vi "ListBox Demo.vi"() -> ()   [LabVIEW 2020]
uses:
  AutoComplete/AutoComplete.lvlib
panel:
  in  "Autohide List?":bool
  in  "Listbox":i32(listbox)
  out "Selection":string
  in  "String":string
  # "This example uses an existing listbox that's part of this VI to show the filtered items."
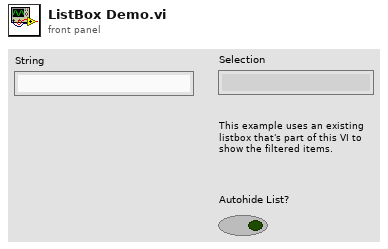
[diagram p1: front panel]
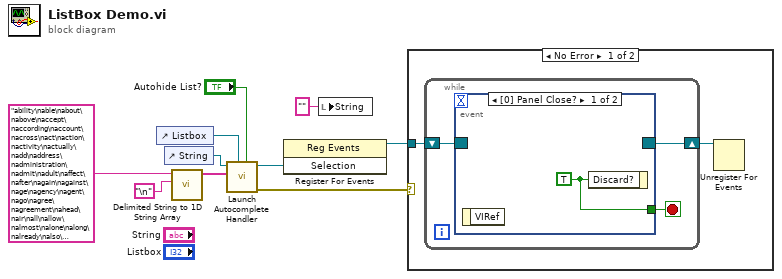
[diagram p0: block diagram]
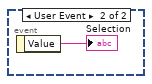
[diagram p2: hidden frame]
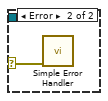
[diagram p3: hidden frame]
diagram:
  n1 = control-ref of="Listbox"() -> (w6:refnum<vi>)
  n2 = control-ref of="String"() -> (w7:refnum<vi>)
  n3 = call <vilib>:"Delimited String to 1D String Array.vi"("delimiter"="\n", "delimited string"="ability\nable\nabout\nabove\naccept\naccording\naccount\nacross\nact\naction\nactivity\nactually\nadd\naddress\nadministration\nadmit\nadult\naffect\nafter\nagain\nagainst\nage\nagency\nagent\nago\nagree\nagreement\nahead\nair\nall\nallow\nalmost\nalone\nalong\nalready\nalso\nalthough\nalways\nAmerican\namong\namount\nanalysis\nand\nanimal\nanother\nanswer\nany\nanyone\nanything\nappear\napply\napproach\narea\nargue\narm\naround\narrive\nart\narticle\nartist\nas\nask\nassume\nat\nattack\nattention\nattorney\naudience\nauthor\nauthority\navailable\navoid\naway\nbaby\nback\nbad\nbag\nball\nbank\nbar\nbase\nbe\nbeat\nbeautiful\nbecause\nbecome\nbed\nbefore\nbegin\nbehavior\nbehind\nbelieve\nbenefit\nbest\nbetter\nbetween\nbeyond\nbig\nbill\nbillion\nbit\nblack\nblood\nblue\nboard\nbody\nbook\nborn\nboth\nbox\nboy\nbreak\nbring\nbrother\nbudget\nbuild\nbuilding\nbusiness\nbut\nbuy\nby\ncall\ncamera\ncampaign\ncan\ncancer\ncandidate\ncapital\ncar\ncard\ncare\ncareer\ncarry\ncase\ncatch\ncause\ncell\ncenter\ncentral\ncentury\ncertain\ncertainly\nchair\nchallenge\nchance\nchange\ncharacter\ncharge\ncheck\nchild\nchoice\nchoose\nchurch\ncitizen\ncity\ncivil\nclaim\nclass\nclear\nclearly\nclose\ncoach\ncold\ncollection\ncollege\ncolor\ncome\ncommercial\ncommon\ncommunity\ncompany\ncompare\ncomputer\nconcern\ncondition\nconference\nCongress\nconsider\nconsumer\ncontain\ncontinue\ncontrol\ncost\ncould\ncountry\ncouple\ncourse\ncourt\ncover\ncreate\ncrime\ncultural\nculture\ncup\ncurrent\ncustomer\ncut\ndark\ndata\ndaughter\nday\ndead\ndeal\ndeath\ndebate\ndecade\ndecide\ndecision\ndeep\ndefense\ndegree\nDemocrat\ndemocratic\ndescribe\ndesign\ndespite\ndetail\ndetermine\ndevelop\ndevelopment\ndie\ndifference\ndifferent\ndifficult\ndinner\ndirection\ndirector\ndiscover\ndiscuss\ndiscussion\ndisease\ndo\ndoctor\ndog\ndoor\ndown\ndraw\ndream\ndrive\ndrop\ndrug\nduring\neach\nearly\neast\neasy\neat\neconomic\neconomy\nedge\neducation\neffect\neffort\neight\neither\nelection\nelse\nemployee\nend\nenergy\nenjoy\nenough\nenter\nentire\nenvironment\nenvironmental\nespecially\nestablish\neven\nevening\nevent\never\nevery\neverybody\neveryone\neverything\nevidence\nexactly\nexample\nexecutive\nexist\nexpect\nexperience\nexpert\nexplain\neye\nface\nfact\nfactor\nfail\nfall\nfamily\nfar\nfast\nfather\nfear\nfederal\nfeel\nfeeling\nfew\nfield\nfight\nfigure\nfill\nfilm\nfinal\nfinally\nfinancial\nfind\nfine\nfinger\nfinish\nfire\nfirm\nfirst\nfish\nfive\nfloor\nfly\nfocus\nfollow\nfood\nfoot\nfor\nforce\nforeign\nforget\nform\nformer\nforward\nfour\nfree\nfriend\nfrom\nfront\nfull\nfund\nfuture\ngame\ngarden\ngas\ngeneral\ngeneration\nget\ngirl\ngive\nglass\ngo\ngoal\ngood\ngovernment\ngreat\ngreen\nground\ngroup\ngrow\ngrowth\nguess\ngun\nguy\nhair\nhalf\nhand\nhang\nhappen\nhappy\nhard\nhave\nhe\nhead\nhealth\nhear\nheart\nheat\nheavy\nhelp\nher\nhere\nherself\nhigh\nhim\nhimself\nhis\nhistory\nhit\nhold\nhome\nhope\nhospital\nhot\nhotel\nhour\nhouse\nhow\nhowever\nhuge\nhuman\nhundred\nhusband\nI\nidea\nidentify\nif\nimage\nimagine\nimpact\nimportant\nimprove\nin\ninclude\nincluding\nincrease\nindeed\nindicate\nindividual\nindustry\ninformation\ninside\ninstead\ninstitution\ninterest\ninteresting\ninternational\ninterview\ninto\ninvestment\ninvolve\nissue\nit\nitem\nits\nitself\njob\njoin\njust\nkeep\nkey\nkid\nkill\nkind\nkitchen\nknow\nknowledge\nland\nlanguage\nlarge\nlast\nlate\nlater\nlaugh\nlaw\nlawyer\nlay\nlead\nleader\nlearn\nleast\nleave\nleft\nleg\nlegal\nless\nlet\nletter\nlevel\nlie\nlife\nlight\nlike\nlikely\nline\nlist\nlisten\nlittle\nlive\nlocal\nlong\nlook\nlose\nloss\nlot\nlove\nlow\nmachine\nmagazine\nmain\nmaintain\nmajor\nmajority\nmake\nman\nmanage\nmanagement\nmanager\nmany\nmarket\nmarriage\nmaterial\nmatter\nmay\nmaybe\nme\nmean\nmeasure\nmedia\nmedical\nmeet\nmeeting\nmember\nmemory\nmention\nmessage\nmethod\nmiddle\nmight\nmilitary\nmillion\nmind\nminute\nmiss\nmission\nmodel\nmodern\nmoment\nmoney\nmonth\nmore\nmorning\nmost\nmother\nmouth\nmove\nmovement\nmovie\nMr\nMrs\nmuch\nmusic\nmust\nmy\nmyself\nname\nnation\nnational\nnatural\nnature\nnear\nnearly\nnecessary\nneed\nnetwork\nnever\nnew\nnews\nnewspaper\nnext\nnice\nnight\nno\nnone\nnor\nnorth\nnot\nnote\nnothing\nnotice\nnow\nn't\nnumber\noccur\nof\noff\noffer\noffice\nofficer\nofficial\noften\noh\noil\nok\nold\non\nonce\none\nonly\nonto\nopen\noperation\nopportunity\noption\nor\norder\norganization\nother\nothers\nour\nout\noutside\nover\nown\nowner\npage\npain\npainting\npaper\nparent\npart\nparticipant\nparticular\nparticularly\npartner\nparty\npass\npast\npatient\npattern\npay\npeace\npeople\nper\nperform\nperformance\nperhaps\nperiod\nperson\npersonal\nphone\nphysical\npick\npicture\npiece\nplace\nplan\nplant\nplay\nplayer\nPM\npoint\npolice\npolicy\npolitical\npolitics\npoor\npopular\npopulation\nposition\npositive\npossible\npower\npractice\nprepare\npresent\npresident\npressure\npretty\nprevent\nprice\nprivate\nprobably\nproblem\nprocess\nproduce\nproduct\nproduction\nprofessional\nprofessor\nprogram\nproject\nproperty\nprotect\nprove\nprovide\npublic\npull\npurpose\npush\nput\nquality\nquestion\nquickly\nquite\nrace\nradio\nraise\nrange\nrate\nrather\nreach\nread\nready\nreal\nreality\nrealize\nreally\nreason\nreceive\nrecent\nrecently\nrecognize\nrecord\nred\nreduce\nreflect\nregion\nrelate\nrelationship\nreligious\nremain\nremember\nremove\nreport\nrepresent\nRepublican\nrequire\nresearch\nresource\nrespond\nresponse\nresponsibility\nrest\nresult\nreturn\nreveal\nrich\nright\nrise\nrisk\nroad\nrock\nrole\nroom\nrule\nrun\nsafe\nsame\nsave\nsay\nscene\nschool\nscience\nscientist\nscore\nsea\nseason\nseat\nsecond\nsection\nsecurity\nsee\nseek\nseem\nsell\nsend\nsenior\nsense\nseries\nserious\nserve\nservice\nset\nseven\nseveral\nsex\nsexual\nshake\nshare\nshe\nshoot\nshort\nshot\nshould\nshoulder\nshow\nside\nsign\nsignificant\nsimilar\nsimple\nsimply\nsince\nsing\nsingle\nsister\nsit\nsite\nsituation\nsix\nsize\nskill\nskin\nsmall\nsmile\nso\nsocial\nsociety\nsoldier\nsome\nsomebody\nsomeone\nsomething\nsometimes\nson\nsong\nsoon\nsort\nsound\nsource\nsouth\nsouthern\nspace\nspeak\nspecial\nspecific\nspeech\nspend\nsport\nspring\nstaff\nstage\nstand\nstandard\nstar\nstart\nstate\nstatement\nstation\nstay\nstep\nstill\nstock\nstop\nstore\nstory\nstrategy\nstreet\nstrong\nstructure\nstudent\nstudy\nstuff\nstyle\nsubject\nsuccess\nsuccessful\nsuch\nsuddenly\nsuffer\nsuggest\nsummer\nsupport\nsure\nsurface\nsystem\ntable\ntake\ntalk\ntask\ntax\nteach\nteacher\nteam\ntechnology\ntelevision\ntell\nten\ntend\nterm\ntest\nthan\nthank\nthat\nthe\ntheir\nthem\nthemselves\nthen\ntheory\nthere\nthese\nthey\nthing\nthink\nthird\nthis\nthose\nthough\nthought\nthousand\nthreat\nthree\nthrough\nthroughout\nthrow\nthus\ntime\nto\ntoday\ntogether\ntonight\ntoo\ntop\ntotal\ntough\ntoward\ntown\ntrade\ntraditional\ntraining\ntravel\ntreat\ntreatment\ntree\ntrial\ntrip\ntrouble\ntrue\ntruth\ntry\nturn\nTV\ntwo\ntype\nunder\nunderstand\nunit\nuntil\nup\nupon\nus\nuse\nusually\nvalue\nvarious\nvery\nvictim\nview\nviolence\nvisit\nvoice\nvote\nwait\nwalk\nwall\nwant\nwar\nwatch\nwater\nway\nwe\nweapon\nwear\nweek\nweight\nwell\nwest\nwestern\nwhat\nwhatever\nwhen\nwhere\nwhether\nwhich\nwhile\nwhite\nwho\nwhole\nwhom\nwhose\nwhy\nwide\nwife\nwill\nwin\nwind\nwindow\nwish\nwith\nwithin\nwithout\nwoman\nwonder\nword\nwork\nworker\nworld\nworry\nwould\nwrite\nwriter\nwrong\nyard\nyeah\nyear\nyes\nyet\nyou\nyoung\nyour\nyourself") -> ("string array"=w1:string[])  [unwired: 9 in]
  n4 = call "Launch Autocomplete Handler.vi"("Autohide ListBox (F)"="Autohide List?", "ListBox Refnum (Popup)"=w6, "Initial Options (Empty)"=w1, "Str Refnum"=w7) -> ("error out"=w8:errorcluster, "Selection"=w4:refnum<user-event>)  [unwired: 4 in, 2 out]
  n5 = register-events(w4) -> (reference out=w3:refnum<event-registration>)  [unwired: 2 in, 1 out]
  n6 = local write "String"("" ("String")) -> ()
  n7 = case shown="No Error" w8 {
    selector: w8 -> [_ w18]
    tunnel: w3 -> [w12 _]
    frame No Error {
      n8 = while {
        shift-right: [w13] -> w11
        shift-left: w12 -> [w14]
        stop <- w15 stop-if-true
        n9 = event shown="[0] Panel Close?" {
          selector: w14 -> [_ _]
          dyn-events: [_ _] -> w13
          timeout: _ -> [_ _]
          tunnel: [w16 _] -> w15
          event Panel Close? {
            w16 = TRUE ("Discard?")
            n10 = event-data() -> ()  [unwired: 1 in, 1 out]
            n11 = event-data("Discard?"=w16) -> ()  [unwired: 1 in, 1 out]
          }
          event User Event {
            n12 = event-data() -> ("Value"=→"Selection":string)  [unwired: 1 in]
          }
        }
      }
      n13 = Unregister For Events(event registration refnum=w11) -> ()  [unwired: 1 in, 1 out]
    }
    frame Error {
      n14 = call <vilib>:"Simple Error Handler.vi"("error in (no error)"=w18) -> ()  [unwired: 4 in, 5 out]
    }
  }
